vi "Word_Set_Table_Align.vi"(0 "Word._Application":refnum<k7>, 1 "start row":i32, 2 "start column":i32, 5 "table":refnum<k7>, 7 "vertical alignment":i32(ring) items=["wdCellAlignVerticalTop"=0, "wdCellAlignVerticalCenter"=1, "wdCellAlignVerticalBottom"=3], 9 "horizontal alignment":i32(ring) items=["wdAlignParagraphLeft"=0, "wdAlignParagraphCenter"=1, "wdAlignParagraphRight"=2, "wdAlignParagraphJustify"=3, "wdAlignParagraphDistribute"=4, "wdAlignParagraphJustifyMed"=5, "wdAlignParagraphJustifyHi"=7, "wdAlignParagraphJustifyLow"=8], 11 "error in":errorcluster, 12 "end row":i32, 13 "end column":i32) -> (15 "error out":errorcluster)   [LabVIEW 2017, in "NI_ReportGenerationToolkit.lvlib"]
uses:
  <vilib>/addons/_office/NI_ReportGenerationToolkit.lvlib
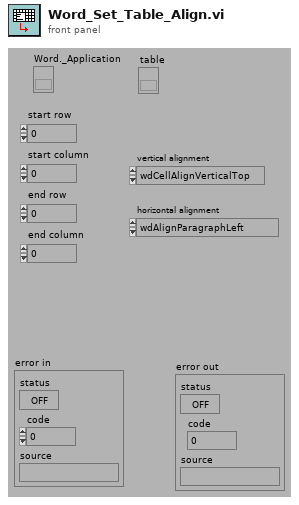
[diagram p1: front panel]
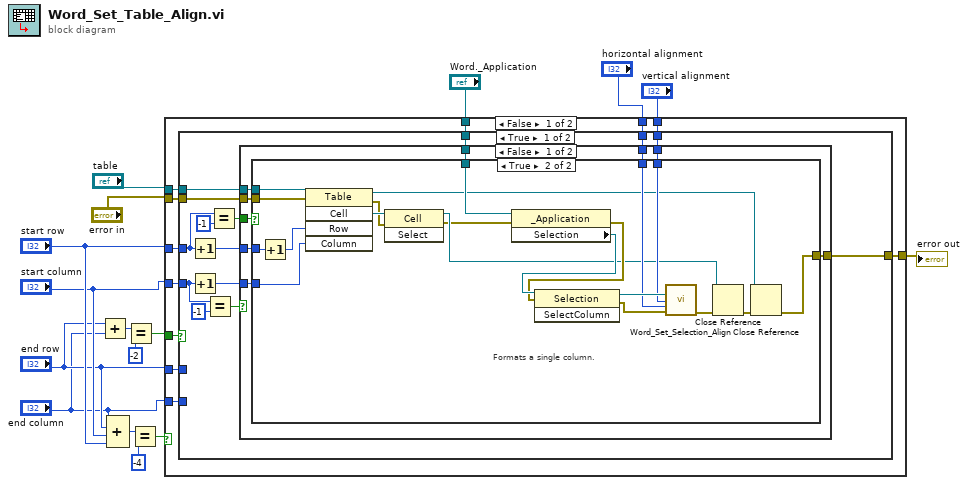
[diagram p0: block diagram]
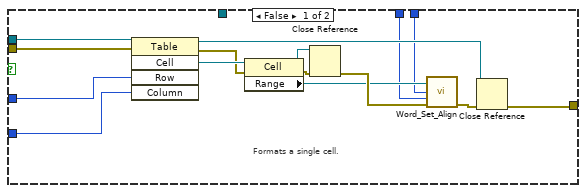
[diagram p2: hidden frame]
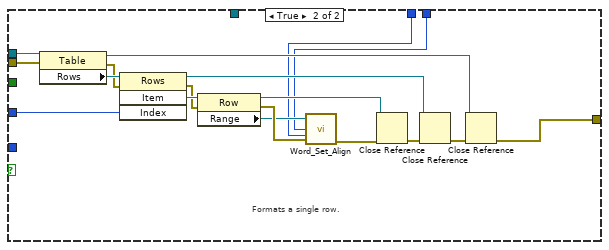
[diagram p3: hidden frame]
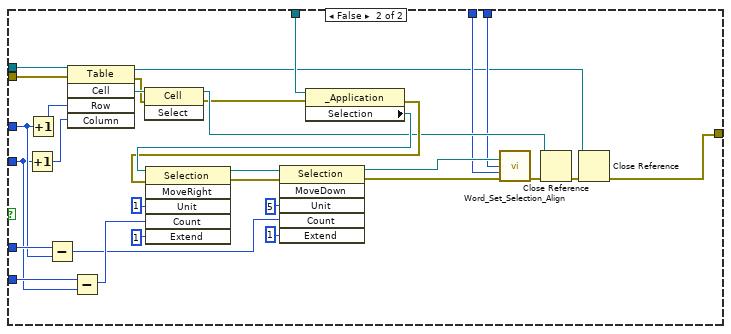
[diagram p4: hidden frame]
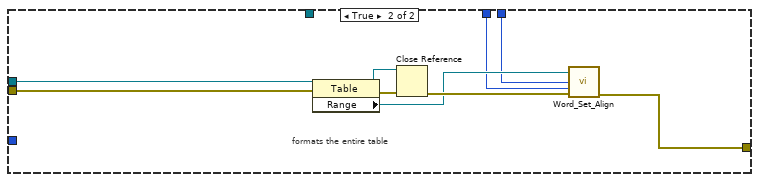
[diagram p5: hidden frame]
diagram:
  n1 = Add(x="end row", y="end column") -> (x+y=w14:i32)
  n2 = Compound Arithmetic op=ADD("end column", "end row", "start column", "start row") -> (w16:i32)
  n3 = Equal?(x=w14, y=-2) -> (x = y?=w6:bool)
  n4 = Equal?(x=w16, y=-4) -> (x = y?=w5:bool)
  n5 = case shown="False" w5 {
    tunnel: "start column" -> [w27 _]
    tunnel: "start row" -> [w26 _]
    tunnel: "end row" -> [w25 _]
    tunnel: "end column" -> [w24 _]
    tunnel: [w23 w135] -> w2
    tunnel: "table" -> [w22 w143]
    tunnel: "error in" -> [w21 w142]
    tunnel: w6 -> [w20 _]
    tunnel: "vertical alignment" -> [w19 w137]
    tunnel: "horizontal alignment" -> [w18 w136]
    tunnel: "Word._Application" -> [w17 _]
    frame False {
      n6 = case shown="True" w20 {
        tunnel: w27 -> [w35 w117]
        tunnel: w26 -> [w32 w118]
        tunnel: w25 -> [_ w120]
        tunnel: w24 -> [_ w119]
        tunnel: [w41 w112] -> w23
        tunnel: w22 -> [w40 w134]
        tunnel: w21 -> [w37 w133]
        tunnel: w19 -> [w30 w108]
        tunnel: w18 -> [w29 w107]
        tunnel: w17 -> [w28 w106]
        frame True {
          n7 = Increment(x=w32) -> (x+1=w39:i32)
          n8 = Increment(x=w35) -> (x+1=w38:i32)
          n9 = Equal?(x=w35, y=-1) -> (x = y?=w36:bool)
          n10 = Equal?(x=w32, y=-1) -> (x = y?=w31:bool)
          n11 = case shown="False" w36 {
            tunnel: [w50 w92] -> w41
            tunnel: w40 -> [w49 w103]
            tunnel: w39 -> [w48 w101]
            tunnel: w38 -> [w47 _]
            tunnel: w37 -> [w46 w97]
            tunnel: w31 -> [w45 _]
            tunnel: w30 -> [w44 w86]
            tunnel: w29 -> [w43 w87]
            tunnel: w28 -> [w42 _]
            frame False {
              n12 = case shown="True" w45 {
                tunnel: [w57 w78] -> w50
                tunnel: w49 -> [w63 w85]
                tunnel: w48 -> [w62 w83]
                tunnel: w47 -> [w61 w82]
                tunnel: w46 -> [w59 w84]
                tunnel: w44 -> [w52 w72]
                tunnel: w43 -> [w51 w71]
                tunnel: w42 -> [_ w70]
                frame False {
                  # "Formats a single cell."
                  n13 = invoke class="Table" method="Cell"(reference=w63, error in=w59, "Row"=w62, "Column"=w61) -> (reference out=w56:refnum<k7>, error out=w58:errorcluster, "Cell"=w60:refnum<k7>)  [unwired: 1 in, 2 out]
                  n14 = property class="Cell"(reference=w60, error in=w58) -> (reference out=w65:refnum<k7>, error out=w64:errorcluster, "Range"=w53:refnum<k7>)
                  n15 = Close Reference(reference=w65, error in (no error)=w64) -> (error out=w55:errorcluster)
                  n16 = call <vilib>:"Word_Set_Align.vi"("Range"=w53, "vertical alignment"=w52, "horizontal alignment"=w51, "error in (no error)"=w55) -> ("error out"=w54:errorcluster)  [unwired: 11 out]
                  n17 = Close Reference(reference=w56, error in (no error)=w54) -> (error out=w57:errorcluster)
                }
                frame True {
                  # "Formats a single column."
                  n18 = Increment(x=w83) -> (x+1=w66:i32)
                  n19 = invoke class="Table" method="Cell"(reference=w85, error in=w84, "Row"=w66, "Column"=w82) -> (reference out=w68:refnum<k7>, error out=w80:errorcluster, "Cell"=w81:refnum<k7>)  [unwired: 1 in, 2 out]
                  n20 = invoke class="Cell" method="Select"(reference=w81, error in=w80) -> (reference out=w69:refnum<k7>, error out=w67:errorcluster)  [unwired: 1 in, 1 out]
                  n21 = property class="_Application"(reference=w70, error in=w67) -> (error out=w76:errorcluster, "Selection"=w77:refnum<k7>)  [unwired: 1 out]
                  n22 = invoke class="Selection" method="SelectColumn"(reference=w77, error in=w76) -> (reference out=w75:refnum<k7>, error out=w74:errorcluster)  [unwired: 1 in, 1 out]
                  n23 = call <vilib>:"Word_Set_Selection_Align.vi"("Word.Selection"=w75, "vertical alignment"=w72, "horizontal alignment"=w71, "error out 2"=w74) -> ("error out"=w73:errorcluster)  [unwired: 1 in, 10 out]
                  n24 = Close Reference(reference=w69, error in (no error)=w73) -> (error out=w79:errorcluster)
                  n25 = Close Reference(reference=w68, error in (no error)=w79) -> (error out=w78:errorcluster)
                }
              }
            }
            frame True {
              # "Formats a single row."
              n26 = property class="Table"(reference=w103, error in=w97) -> (reference out=w91:refnum<k7>, error out=w99:errorcluster, "Rows"=w102:refnum<k7>)
              n27 = invoke class="Rows" method="Item"(reference=w102, error in=w99, "Index"=w101) -> (reference out=w94:refnum<k7>, error out=w98:errorcluster, "Item"=w100:refnum<k7>)  [unwired: 1 in, 1 out]
              n28 = property class="Row"(reference=w100, error in=w98) -> (reference out=w95:refnum<k7>, error out=w90:errorcluster, "Range"=w88:refnum<k7>)
              n29 = call <vilib>:"Word_Set_Align.vi"("Range"=w88, "vertical alignment"=w86, "horizontal alignment"=w87, "error in (no error)"=w90) -> ("error out"=w89:errorcluster)  [unwired: 11 out]
              n30 = Close Reference(reference=w95, error in (no error)=w89) -> (error out=w96:errorcluster)
              n31 = Close Reference(reference=w94, error in (no error)=w96) -> (error out=w93:errorcluster)
              n32 = Close Reference(reference=w91, error in (no error)=w93) -> (error out=w92:errorcluster)
            }
          }
        }
        frame False {
          n33 = Increment(x=w117) -> (x+1=w131:i32)
          n34 = Increment(x=w118) -> (x+1=w132:i32)
          n35 = Subtract(x=w120, y=w118) -> (x-y=w115:i32)
          n36 = invoke class="Table" method="Cell"(reference=w134, error in=w133, "Row"=w132, "Column"=w131) -> (reference out=w104:refnum<k7>, error out=w129:errorcluster, "Cell"=w130:refnum<k7>)  [unwired: 1 in, 2 out]
          n37 = Subtract(x=w119, y=w117) -> (x-y=w116:i32)
          n38 = invoke class="Cell" method="Select"(reference=w130, error in=w129) -> (reference out=w113:refnum<k7>, error out=w105:errorcluster)  [unwired: 1 in, 1 out]
          n39 = property class="_Application"(reference=w106, error in=w105) -> (error out=w127:errorcluster, "Selection"=w128:refnum<k7>)  [unwired: 1 out]
          n40 = invoke class="Selection" method="MoveRight"(reference=w128, error in=w127, "Unit"=1, "Count"=w116, "Extend"=1) -> (reference out=w124:refnum<k7>, error out=w123:errorcluster)  [unwired: 1 in, 4 out]
          n41 = invoke class="Selection" method="MoveDown"(reference=w124, error in=w123, "Unit"=5, "Count"=w115, "Extend"=1) -> (reference out=w109:refnum<k7>, error out=w111:errorcluster)  [unwired: 1 in, 4 out]
          n42 = call <vilib>:"Word_Set_Selection_Align.vi"("Word.Selection"=w109, "vertical alignment"=w108, "horizontal alignment"=w107, "error out 2"=w111) -> ("error out"=w110:errorcluster)  [unwired: 1 in, 10 out]
          n43 = Close Reference(reference=w113, error in (no error)=w110) -> (error out=w114:errorcluster)
          n44 = Close Reference(reference=w104, error in (no error)=w114) -> (error out=w112:errorcluster)
        }
      }
    }
    frame True {
      # "formats the entire table"
      n45 = property class="Table"(reference=w143, error in=w142) -> (reference out=w140:refnum<k7>, error out=w141:errorcluster, "Range"=w138:refnum<k7>)
      n46 = Close Reference(reference=w140, error in (no error)=w141) -> (error out=w139:errorcluster)
      n47 = call <vilib>:"Word_Set_Align.vi"("Range"=w138, "vertical alignment"=w137, "horizontal alignment"=w136, "error in (no error)"=w139) -> ("error out"=w135:errorcluster)  [unwired: 11 out]
    }
  }
  "error out" <- w2
